vi "trajetoria do centro.vi"(8 "Color":u32(colorbox)=6618880, 9 "pontos\ninterpolados":cluster{"X":dbl, "Y":dbl}[](array[cluster]), 10 "target size":cluster{"sx":i32, "sy":i32}, 11 "Refnum in":T1) -> (3 "Refnum out":T1)   [LabVIEW 2016]
uses:
  <vilib>/vision/Image Controls.llb/IMAQ Image.ctl
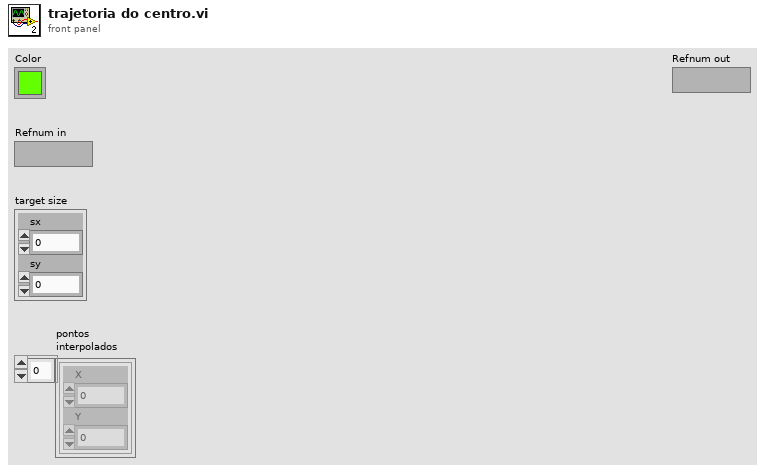
[diagram p1: front panel]
types:
  T1 = typedef "IMAQ Image.ctl" = refnum<image>
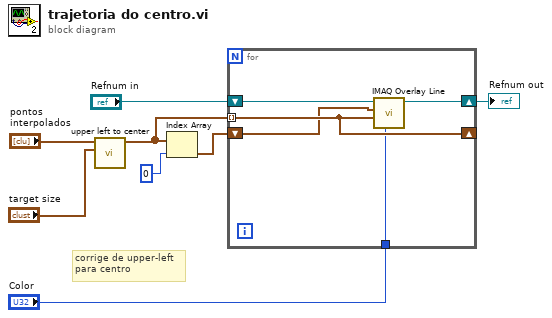
[diagram p0: block diagram]
diagram:
  # "corrige de upper-left\npara centro"
  n1 = call "upper left to center.vi"("target size"="target size", "ponto in"="pontos\ninterpolados") -> ("ponto out"=w4:cluster{"X":dbl, "Y":dbl}[])  [unwired: 9 in]
  n2 = Index Array(array=w4, index=0) -> (element=w7:cluster{"X":dbl, "Y":dbl})
  n3 = for {
    shift-right: [w13] -> _
    shift-left: w7 -> [w11]
    tunnel: w4 -> [w13] mode=indexing
    tunnel: "Color" -> [w10]
    shift-right: [w9] -> w1
    shift-left: "Refnum in" -> [w12]
    n4 = call "IMAQ Overlay Line"("Color"=w10, "End Point"=w13, "Start Point"=w11, "Image"=w12) -> ("Image Out"=w9:T1)  [unwired: 6 in, 1 out]
  }
  "Refnum out" <- w1
